vi "I2C Traffic Monitor.vi"(0 "channel i2c io":T2, 1 "reset":bool) -> (4 "i2c monitor":T1 {"monitor word" format="%.0x"})   [LabVIEW 2020, in "GettingStarted_Common_148X_FPGA.lvlib"]
uses:
  GettingStarted_Common_148X_FPGA.lvlib
  Types/I2C IO.ctl
  <instrlib>/FlexRIO/API/FPGA/v1/IO/NI148x/i2c monitor.ctl
  <instrlib>/FlexRIO/API/FPGA/v1/IO/NI148x/Single I2C In.ctl
  <vilib>/rvi/eio/common/nirviEmuTemplateMethod_errors.vi
  <vilib>/eio/EIONode/EIONode.xnode
  <instrlib>/FlexRIO/API/FPGA/v1/IO/NI148x/FlexRIO 148x FPGA v1.lvlib
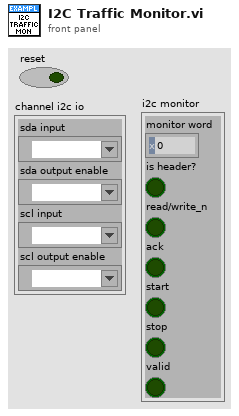
[diagram p1: front panel]
types:
  T1 = typedef "FlexRIO 148x FPGA v1.lvlib/i2c monitor.ctl" = cluster{"monitor word":u8, "is header?":bool, "read/write_n":bool, "ack":bool, "start":bool, "stop":bool, "valid":bool}
  T2 = typedef "GettingStarted_Common_148X_FPGA.lvlib/I2C IO.ctl" = cluster{"sda input":refnum<k21>, "sda output enable":refnum<k21>, "scl input":refnum<k21>, "scl output enable":refnum<k21>}
  T3 = typedef "FlexRIO 148x FPGA v1.lvlib/Single I2C In.ctl" = cluster{"SCL_I":bool, "SDA_I":bool}
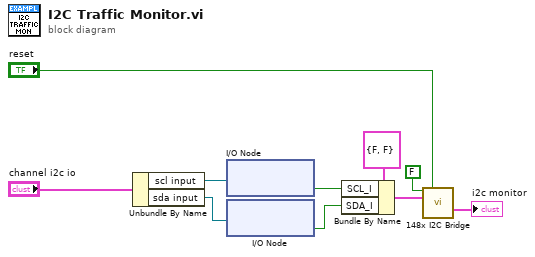
[diagram p0: block diagram]
diagram:
  n1 = Unbundle By Name("channel i2c io") -> ("scl input"=w7:refnum<k21>, "sda input"=w5:refnum<k21>)
  n2 = xnode "I/O Node"("FPGA I/O In"=w7) -> ("I/O Item"=w3:bool)  [unwired: 1 out]
  n3 = xnode "I/O Node"("FPGA I/O In"=w5) -> ("I/O Item"=w4:bool)  [unwired: 1 out]
  n4 = Bundle By Name(cluster=T3 {"SCL_I"=FALSE, "SDA_I"=FALSE} ("i2c 0 in"), "SCL_I"=w3, "SDA_I"=w4) -> (w6:T3)
  n5 = call <instrlib>:"148x I2C Bridge.vi"("enable tap bridge"=FALSE ("enable i2c tap bridge"), "reset"="reset", "i2c 0 in"=w6) -> ("i2c monitor"=→"i2c monitor":T1)  [unwired: 10 in, 2 out]
